vi "Branding.vi"(8 "error in":errorcluster, 11 "This VI":refnum<vi>) -> ()   [LabVIEW 2020, in "ConstantErrorsMaker.lvlib"]
uses:
  ConstantErrorsMaker.lvlib
  <vilib>/Utility/miscctls.llb/LVRowAndColumnTypeDef.ctl
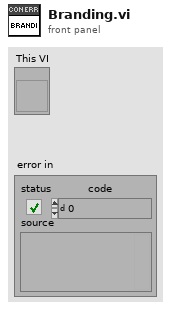
[diagram p1: front panel]
types:
  T1 = typedef "ConstantErrorsMaker.lvlib/Style--cluster.ctl" = cluster{"Gris Obscuro Azul":u32, "Gris Medio Azul":u32, "Gris Claro Azul":u32, "Amarillo":u32, "Text color":u32, "Transparent":u32, "Fuente":string, "Text.Font:Size":u32}
  T2 = typedef "LVRowAndColumnTypeDef.ctl" = cluster{"Row":i32, "Column":i32}
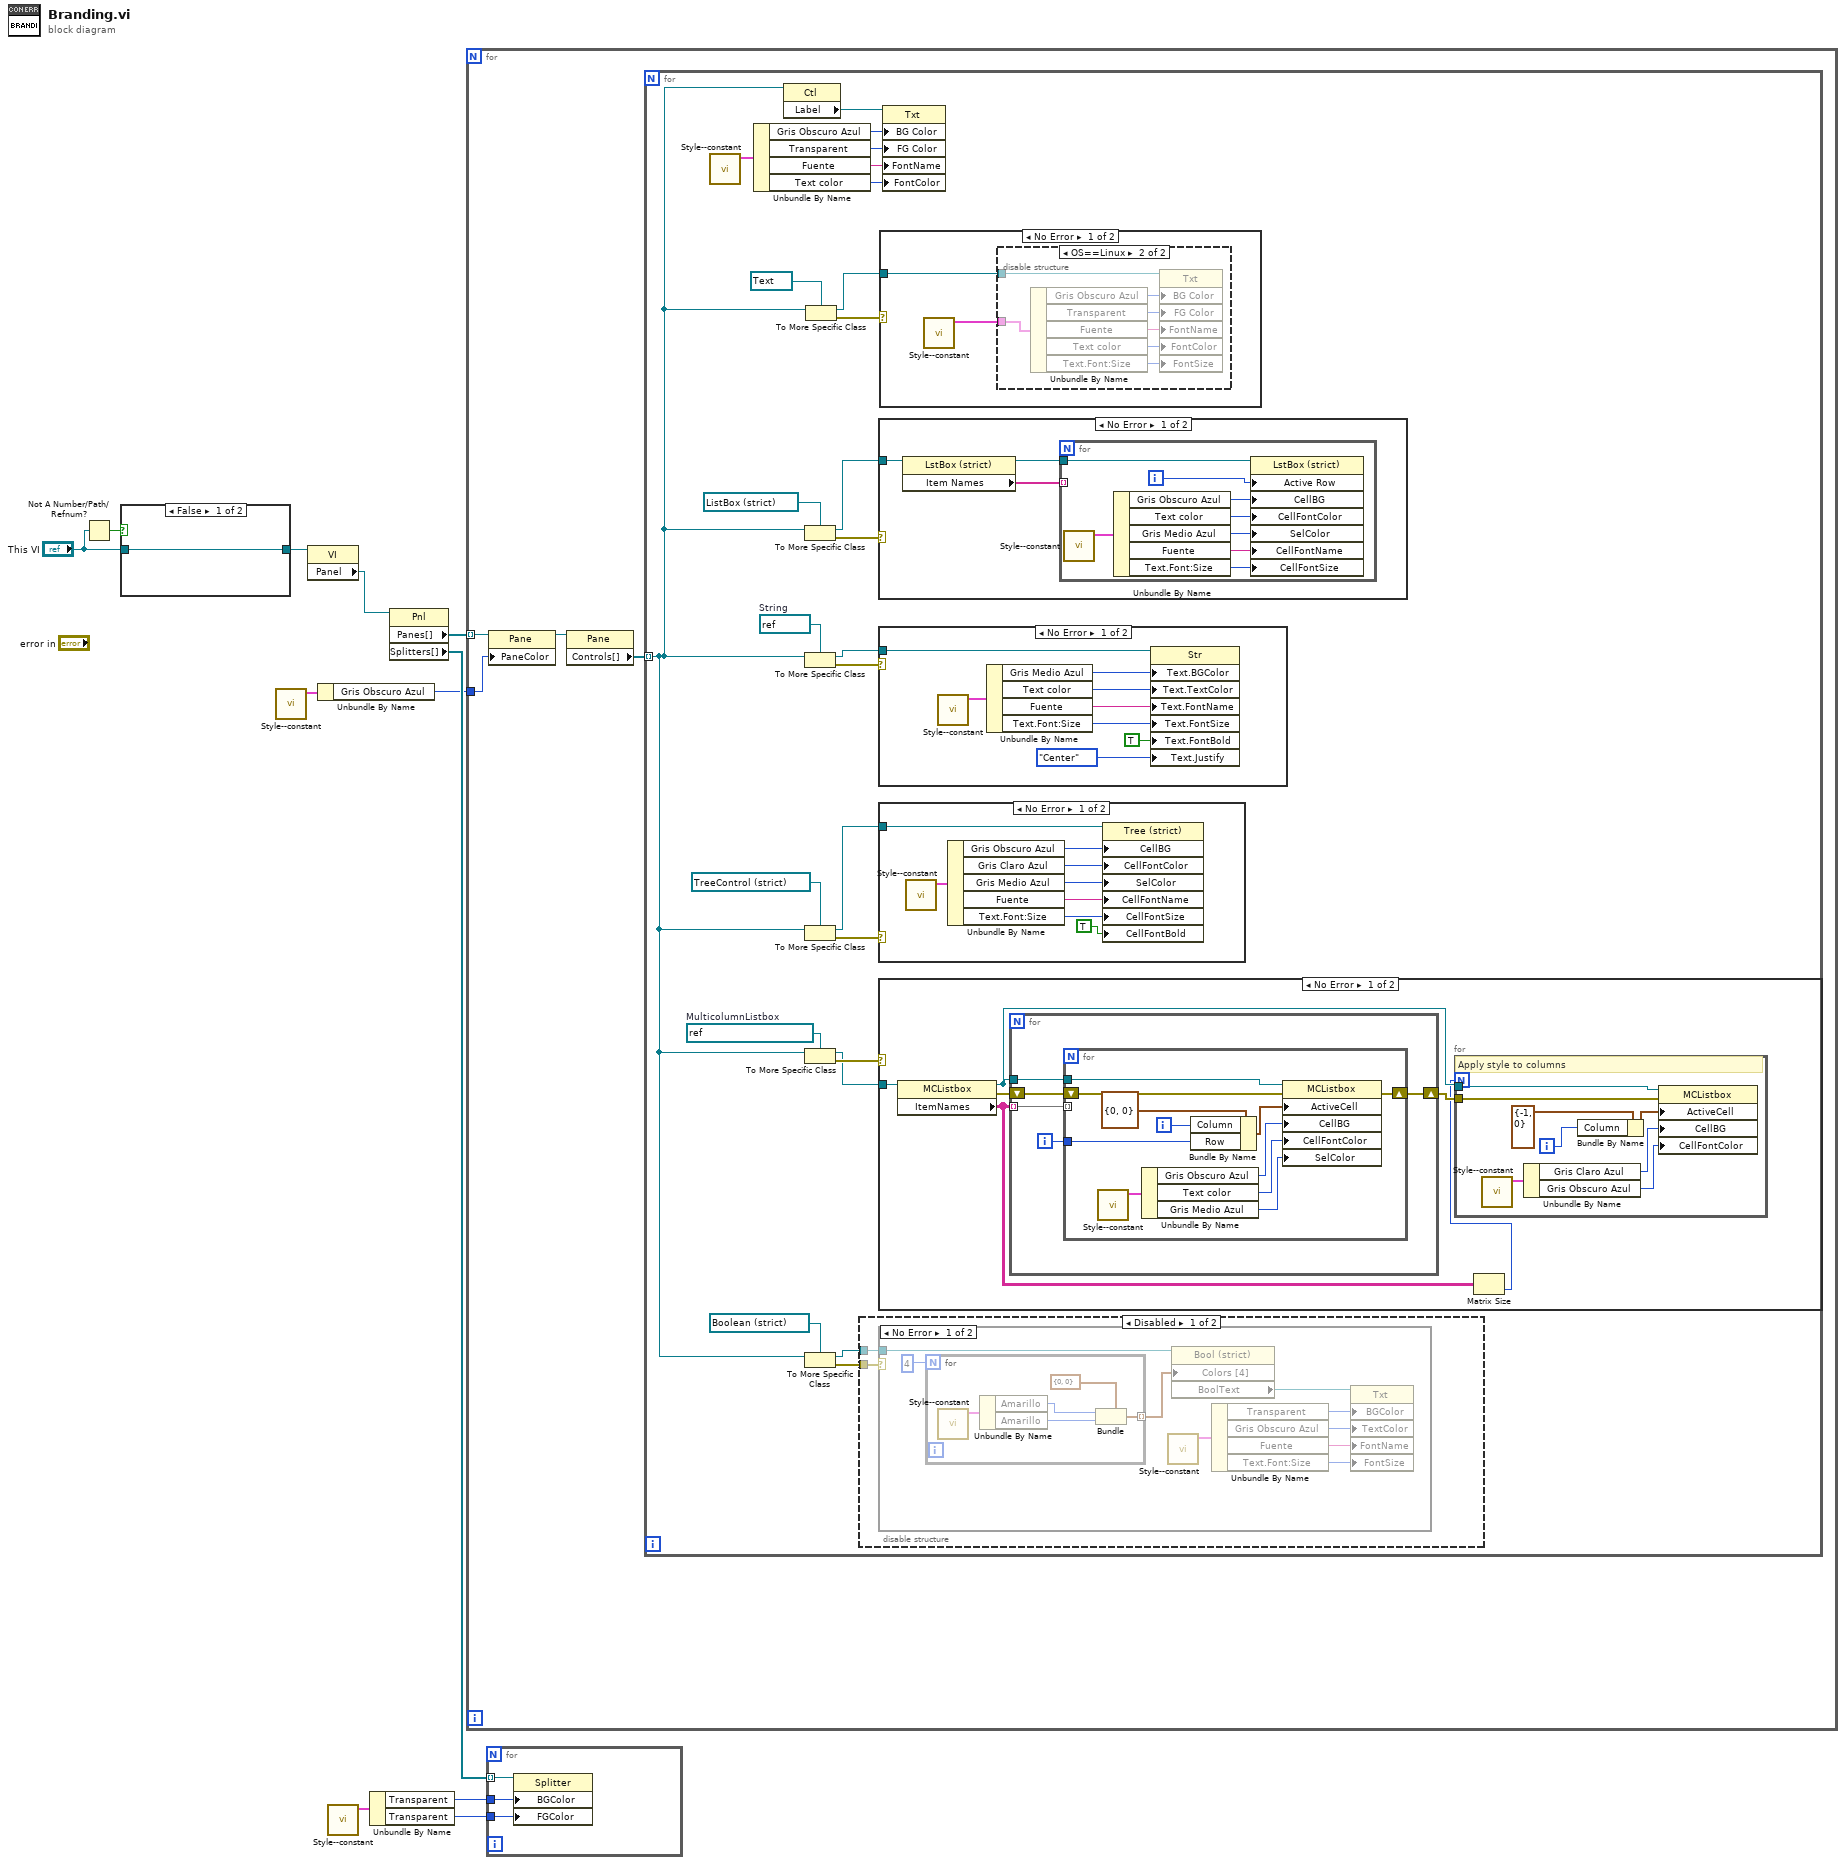
[diagram p0: block diagram]
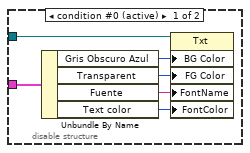
[diagram p4: hidden frame]
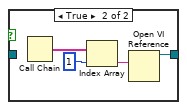
[diagram p10: hidden frame]
diagram:
  n1 = Not A Number/Path/Refnum?(number/path/refnum="This VI") -> (NaN/Path/Refnum?=w11:bool)
  n2 = case shown="False" w11 {
    tunnel: [w12 w13] -> w9
    tunnel: "This VI" -> [w12 _]
    frame False {
    }
    frame True {
      n3 = Call Chain() -> (call chain=w16:string[])
      n4 = Index Array(array=w16, index=1) -> (element=w14:string)
      n5 = Open VI Reference(vi path=w14) -> (vi reference=w13:refnum<vi>)  [unwired: 5 in, 1 out]
    }
  }
  n6 = call "Style--constant.vi"() -> ("Style"=w2:T1)  [unwired: 11 in]
  n7 = property class="VI"(reference=w9) -> ("Panel"=w8:refnum<vi>)  [unwired: 1 in, 2 out]
  n8 = Unbundle By Name(w2) -> ("Gris Obscuro Azul"=w1:u32)
  n9 = call "Style--constant.vi"() -> ("Style"=w5:T1)  [unwired: 11 in]
  n10 = Unbundle By Name(w5) -> ("Transparent"=w4:u32, "Transparent"=w3:u32)
  n11 = property class="Pnl"(reference=w8) -> ("Panes[]"=w7:refnum<vi>[], "Splitters[]"=w6:refnum<vi>[])  [unwired: 1 in, 2 out]
  n12 = for {
    tunnel: w7 -> [w20] mode=indexing
    tunnel: w1 -> [w17]
    n13 = property class="Pane"(reference=w20, "PaneColor"=w17) -> (reference out=w19:refnum<vi>)  [unwired: 1 in, 1 out]
    n14 = property class="Pane"(reference=w19) -> ("Controls[]"=w18:refnum<vi>[])  [unwired: 1 in, 2 out]
    n15 = for {
      tunnel: w18 -> [w22] mode=indexing
      w34 = refnum<vi> refnum  # String
      w35 = refnum<vi> refnum  # MulticolumnListbox
      n16 = call "Style--constant.vi"() -> ("Style"=w31:T1)  [unwired: 11 in]
      n17 = Unbundle By Name(w31) -> ("Gris Obscuro Azul"=w30:u32, "Transparent"=w27:u32, "Fuente"=w29:string, "Text color"=w28:u32)
      n18 = property class="Ctl"(reference=w22) -> ("Label"=w32:refnum<vi>)  [unwired: 1 in, 2 out]
      n19 = To More Specific Class(target class=refnum<vi> refnum ("Project history"), reference=w22) -> (specific class reference=w37:refnum<vi>, error out=w43:errorcluster)  [unwired: 1 in]
      n20 = To More Specific Class(target class=w34, reference=w22) -> (specific class reference=w33:refnum<vi>, error out=w41:errorcluster)  [unwired: 1 in]
      n21 = To More Specific Class(target class=refnum<vi> refnum ("Tree Control"), reference=w22) -> (specific class reference=w38:refnum<vi>, error out=w44:errorcluster)  [unwired: 1 in]
      n22 = To More Specific Class(target class=w35, reference=w22) -> (specific class reference=w36:refnum<vi>, error out=w42:errorcluster)  [unwired: 1 in]
      n23 = To More Specific Class(target class=refnum<vi> refnum ("Scan All"), reference=w22) -> (specific class reference=w39:refnum<vi>, error out=w45:errorcluster)  [unwired: 1 in]
      n24 = To More Specific Class(target class=refnum<vi> refnum ("Project history"), reference=w22) -> (specific class reference=w23:refnum<vi>, error out=w40:errorcluster)  [unwired: 1 in]
      n25 = disable-structure shown="Disabled" {
        disable-tunnel: w45 -> [w47 _]
        disable-tunnel: w39 -> [w46 _]
        frame Disabled {
          n26 = case shown="No Error" w47 {
            tunnel: w46 -> [w50 _]
            frame No Error {
              n27 = for {
                N: 4 -> [_]
                tunnel: [w60] -> w55 mode=indexing
                n28 = call "Style--constant.vi"() -> ("Style"=w59:T1)  [unwired: 11 in]
                n29 = Unbundle By Name(w59) -> ("Amarillo"=w57:u32, "Amarillo"=w58:u32)
                n30 = Bundle(cluster=cluster{u32, u32} {0, 0} ("Colors [4]"), w57, w58) -> (w60:cluster{u32, u32})
              }
              n31 = call "Style--constant.vi"() -> ("Style"=w53:T1)  [unwired: 11 in]
              n32 = property class="Bool (strict)"(reference=w50, "Colors [4]"=w55) -> ("BoolText"=w56:refnum<vi>)  [unwired: 1 in, 2 out]
              n33 = Unbundle By Name(w53) -> ("Transparent"=w52:u32, "Gris Obscuro Azul"=w51:u32, "Fuente"=w49:string, "Text.Font:Size"=w48:u32)
              n34 = property class="Txt"(reference=w56, "BGColor"=w52, "TextColor"=w51, "FontName"=w49, "FontSize"=w48) -> ()  [unwired: 1 in, 2 out]
            }
            frame Error {
            }
          }
        }
        frame Enabled {
        }
      }
      n35 = case shown="No Error" w43 {
        tunnel: w37 -> [w125 _]
        frame No Error {
          n36 = property class="LstBox (strict)"(reference=w125) -> (reference out=w124:refnum<vi>, "Item Names"=w123:string[])  [unwired: 1 in, 1 out]
          n37 = for {
            tunnel: w124 -> [w128]
            tunnel: w123 -> [_] mode=indexing
            i -> [w126]
            n38 = call "Style--constant.vi"() -> ("Style"=w133:T1)  [unwired: 11 in]
            n39 = Unbundle By Name(w133) -> ("Gris Obscuro Azul"=w127:u32, "Text color"=w132:u32, "Gris Medio Azul"=w131:u32, "Fuente"=w130:string, "Text.Font:Size"=w129:u32)
            n40 = property class="LstBox (strict)"(reference=w128, "Active Row"=w126, "CellBG"=w127, "CellFontColor"=w132, "SelColor"=w131, "CellFontName"=w130, "CellFontSize"=w129) -> ()  [unwired: 1 in, 2 out]
          }
        }
        frame Error {
        }
      }
      n41 = case shown="No Error" w41 {
        tunnel: w33 -> [w84 _]
        frame No Error {
          n42 = call "Style--constant.vi"() -> ("Style"=w83:T1)  [unwired: 11 in]
          n43 = Unbundle By Name(w83) -> ("Gris Medio Azul"=w82:u32, "Text color"=w81:u32, "Fuente"=w80:string, "Text.Font:Size"=w79:u32)
          n44 = property class="Str"(reference=w84, "Text.BGColor"=w82, "Text.TextColor"=w81, "Text.FontName"=w80, "Text.FontSize"=w79, "Text.FontBold"=TRUE ("Text.Font:Bold"), "Text.Justify"=enum16{"Left", "Center", "Right"}."Center" ("Text.Justification")) -> ()  [unwired: 1 in, 2 out]
        }
        frame Error {
        }
      }
      n45 = case shown="No Error" w44 {
        tunnel: w38 -> [w117 _]
        frame No Error {
          n46 = call "Style--constant.vi"() -> ("Style"=w122:T1)  [unwired: 11 in]
          n47 = Unbundle By Name(w122) -> ("Gris Obscuro Azul"=w121:u32, "Gris Claro Azul"=w120:u32, "Gris Medio Azul"=w119:u32, "Fuente"=w118:string, "Text.Font:Size"=w116:u32)
          n48 = property class="Tree (strict)"(reference=w117, "CellBG"=w121, "CellFontColor"=w120, "SelColor"=w119, "CellFontName"=w118, "CellFontSize"=w116, "CellFontBold"=TRUE ("Active Cell:Cell Font:Bold")) -> ()  [unwired: 1 in, 2 out]
        }
        frame Error {
        }
      }
      n49 = case shown="No Error" w42 {
        tunnel: w36 -> [w88 _]
        frame No Error {
          n50 = property class="MCListbox"(reference=w88) -> (reference out=w87:refnum<vi>, error out=w90:errorcluster, "ItemNames"=w86:string[][])  [unwired: 1 in]
          n51 = for {
            tunnel: w87 -> [w101]
            tunnel: w86 -> [w99] mode=indexing
            shift-right: [w102] -> w89
            shift-left: w90 -> [w103]
            i -> [w100]
            n52 = for {
              tunnel: w101 -> [w109]
              tunnel: w100 -> [w104]
              tunnel: w99 -> [_] mode=indexing
              shift-right: [w113] -> w102
              shift-left: w103 -> [w114]
              i -> [w105]
              n53 = call "Style--constant.vi"() -> ("Style"=w112:T1)  [unwired: 11 in]
              n54 = Unbundle By Name(w112) -> ("Gris Obscuro Azul"=w108:u32, "Text color"=w111:u32, "Gris Medio Azul"=w110:u32)
              n55 = Bundle By Name(cluster=T2 {"Row"=0, "Column"=0} ("Active Cell:Active Cell"), "Column"=w105, "Row"=w104) -> (w106:T2)
              n56 = property class="MCListbox"(reference=w109, error in=w114, "ActiveCell"=w106, "CellBG"=w108, "CellFontColor"=w111, "SelColor"=w110) -> (error out=w113:errorcluster)  [unwired: 1 out]
            }
          }
          n57 = Matrix Size(0:w86) -> (2:w85:i32)  [unwired: 1 out]
          n58 = for {
            N: w85 -> [_]
            tunnel: w89 -> [w98]
            tunnel: w87 -> [w97]
            i -> [w91]
            # "Apply style to columns"
            n59 = call "Style--constant.vi"() -> ("Style"=w95:T1)  [unwired: 11 in]
            n60 = Unbundle By Name(w95) -> ("Gris Claro Azul"=w94:u32, "Gris Obscuro Azul"=w93:u32)
            n61 = Bundle By Name(cluster=T2 {"Row"=-1, "Column"=0} ("Active Cell:Active Cell"), "Column"=w91) -> (w92:T2)
            n62 = property class="MCListbox"(reference=w97, error in=w98, "ActiveCell"=w92, "CellBG"=w94, "CellFontColor"=w93) -> ()  [unwired: 2 out]
          }
        }
        frame Error {
        }
      }
      n63 = case shown="No Error" w40 {
        tunnel: w23 -> [w62 _]
        frame No Error {
          n64 = call "Style--constant.vi"() -> ("Style"=w63:T1)  [unwired: 11 in]
          n65 = disable-structure shown="OS==Linux" {
            disable-tunnel: w63 -> [w69 w76]
            disable-tunnel: w62 -> [w64 w71]
            frame condition #0 (active) {
              n66 = Unbundle By Name(w69) -> ("Gris Obscuro Azul"=w68:u32, "Transparent"=w65:u32, "Fuente"=w67:string, "Text color"=w66:u32)
              n67 = property class="Txt"(reference=w64, "BG Color"=w68, "FG Color"=w65, "FontName"=w67, "FontColor"=w66) -> ()  [unwired: 1 in, 2 out]
            }
            frame condition #1 {
              n68 = Unbundle By Name(w76) -> ("Gris Obscuro Azul"=w75:u32, "Transparent"=w72:u32, "Fuente"=w74:string, "Text color"=w73:u32, "Text.Font:Size"=w70:u32)
              n69 = property class="Txt"(reference=w71, "BG Color"=w75, "FG Color"=w72, "FontName"=w74, "FontColor"=w73, "FontSize"=w70) -> ()  [unwired: 1 in, 2 out]
            }
          }
        }
        frame Error {
        }
      }
      n70 = property class="Txt"(reference=w32, "BG Color"=w30, "FG Color"=w27, "FontName"=w29, "FontColor"=w28) -> ()  [unwired: 1 in, 2 out]
    }
  }
  n71 = for {
    tunnel: w6 -> [w136] mode=indexing
    tunnel: w4 -> [w135]
    tunnel: w3 -> [w134]
    n72 = property class="Splitter"(reference=w136, "BGColor"=w135, "FGColor"=w134) -> ()  [unwired: 1 in, 2 out]
  }
